vi "Get or Add CellStyleFormats.vi"(8 "error in":errorcluster, 11 "SpreadsheetDoc in":refnum<k24>) -> (0 "error out":errorcluster, 2 "CellStyleFormats":refnum<k24>, 3 "SpreadsheetDoc out":refnum<k24>)   [LabVIEW 2019, in "Open Xml.lvlib"]
uses:
  Open Xml.lvlib
  D:/git/Open-Xml-LabVIEW/Source/DocumentFormat.OpenXml.dll
  DocumentFormat.OpenXml.dll
  D:/git/Open-Xml-LabVIEW/Source/DocumentFormat.OpenXml.Framework.dll
  DocumentFormat.OpenXml.Framework.dll
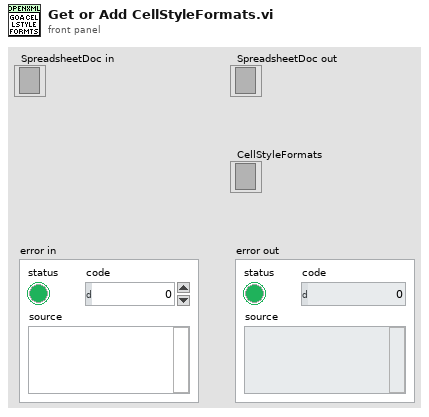
[diagram p1: front panel]
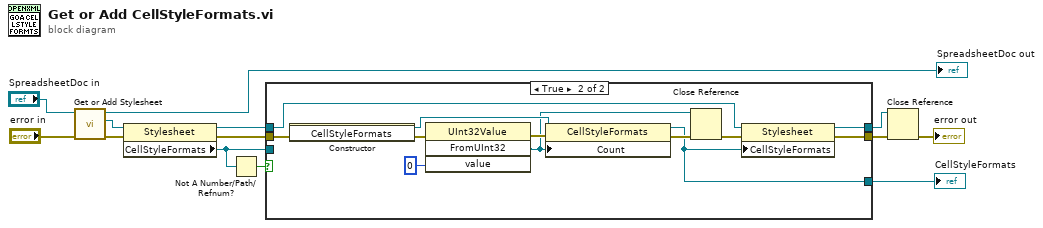
[diagram p0: block diagram]
diagram:
  n1 = call "Get or Add Stylesheet.vi"("error in"="error in", "SpreadsheetDoc in"="SpreadsheetDoc in") -> ("error out"=w9:errorcluster, "Stylesheet"=w7:refnum<k24>, "SpreadsheetDoc out"=→"SpreadsheetDoc out":refnum<k24>)  [unwired: 7 in]
  n2 = property class="Stylesheet"(reference=w7, error in=w9) -> (reference out=w5:refnum<k24>, error out=w12:errorcluster, "CellStyleFormats"=w4:refnum<k24>)
  n3 = Not A Number/Path/Refnum?(number/path/refnum=w4) -> (NaN/Path/Refnum?=w10:bool)
  n4 = case shown="True" w10 {
    tunnel: w12 -> [w16 w28]
    tunnel: [w16 w27] -> w11
    tunnel: w5 -> [w14 w26]
    tunnel: w4 -> [w15 _]
    tunnel: [w15 w18] -> w3
    tunnel: [w14 w17] -> w1
    frame False {
    }
    frame True {
      n5 = constructor class="CellStyleFormats"(error in=w28) -> (reference out=w20:refnum<k24>, error out=w22:errorcluster)  [unwired: 2 in, 1 out]
      n6 = invoke class="UInt32Value" method="FromUInt32"(error in=w22, "value"=u32 0) -> (error out=w21:errorcluster, "FromUInt32"=w19:refnum<k24>)  [unwired: 2 in, 2 out]
      n7 = property class="CellStyleFormats"(reference=w20, error in=w21, "Count"=w19) -> (reference out=w18:refnum<k24>, error out=w25:errorcluster)
      n8 = Close Reference(reference=w19, error in (no error)=w25) -> (error out=w23:errorcluster)
      n9 = property class="Stylesheet"(reference=w26, error in=w23, "CellStyleFormats"=w18) -> (reference out=w17:refnum<k24>, error out=w27:errorcluster)
    }
  }
  "CellStyleFormats" <- w3
  n10 = Close Reference(reference=w1, error in (no error)=w11) -> (error out=→"error out":errorcluster)
